vi "Value High.vi"(1 "In":bool) -> (0 "Out":bool)   [LabVIEW 2016]
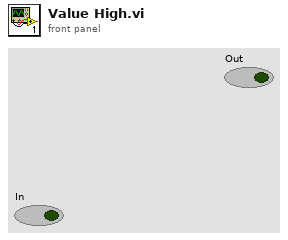
[diagram p1: front panel]
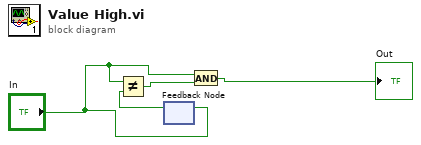
[diagram p0: block diagram]
diagram:
  n1 = feedback #1() -> (w3:bool)  [unwired: 1 in]
  n2 = Not Equal?(x="In", y=w3) -> (x != y?=w4:bool)
  n3 = feedback-in #1("In") -> ()
  n4 = And(x="In", y=w4) -> (x .and. y?=→"Out":bool)
